vi "test - start with default path.vi"(8 "error in (no error)":errorcluster, 11 "TestCase in":refnum<class "testcase-csm-file-logger.lvclass">) -> (0 "error out":errorcluster, 3 "TestCase out":refnum<class "testcase-csm-file-logger.lvclass">)   [LabVIEW 2017, in "testcase-csm-file-logger.lvclass"]
uses:
  testcase-csm-file-logger.lvclass
  <vilib>/addons/_JKI Toolkits/VI Tester/TestCase.llb/TestCase.lvclass
  user.lib/_NEVSTOP/Communicable State Machine(CSM)/addons/Logger/CSM File Logger.lvlib
  C:/Program Files (x86)/National Instruments/LabVIEW 2017/vi.lib/addons/_JKI Toolkits/VI Tester/TestCase.llb/TestCase.lvclass
panel:
  out "LogFile":path
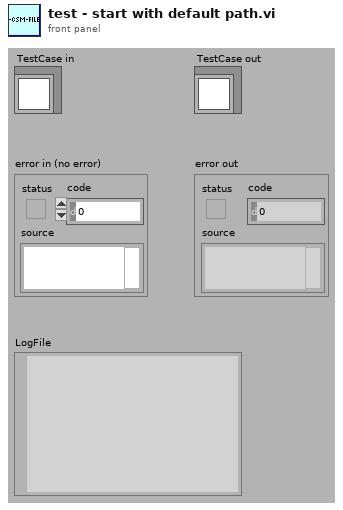
[diagram p1: front panel]
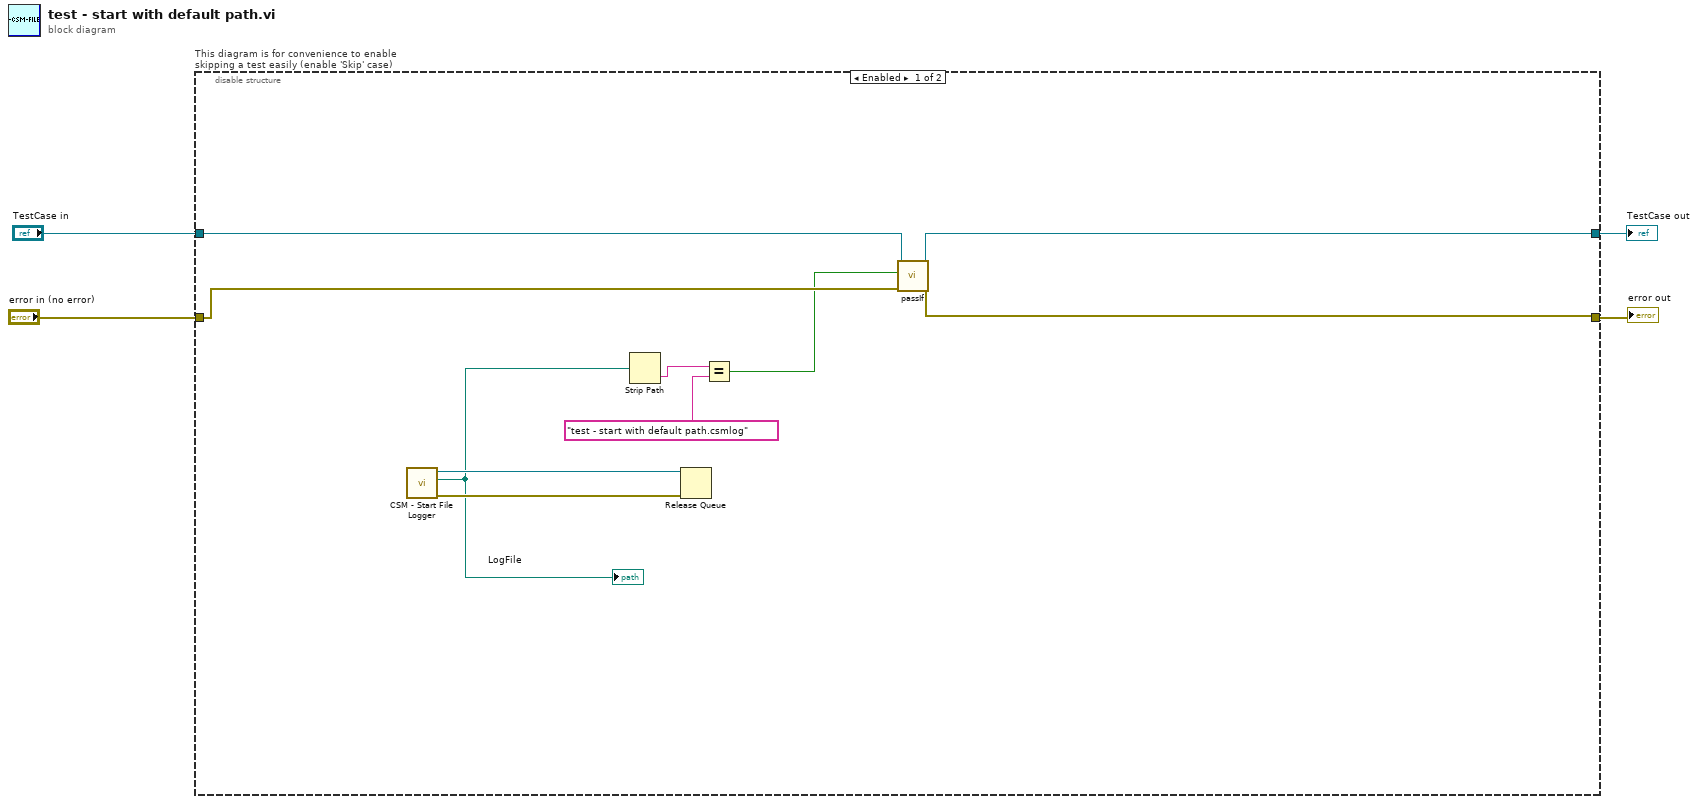
[diagram p0: block diagram]
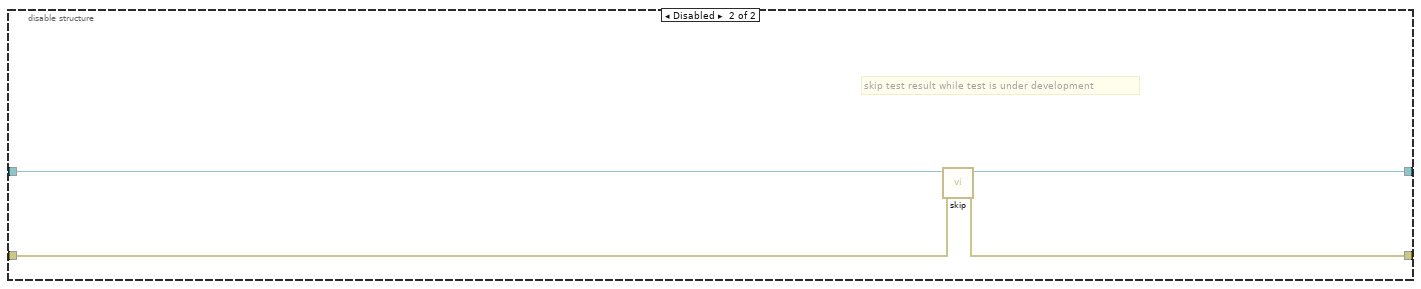
[diagram p2: hidden frame]
diagram:
  n1 = disable-structure "This diagram is for convenience to enable skipping a test easily (enable 'Skip' case)" shown="Enabled" {
    disable-tunnel: "TestCase in" -> [w14 w18]
    disable-tunnel: [w13 w16] -> w1
    disable-tunnel: [w12 w17] -> w3
    disable-tunnel: "error in (no error)" -> [w11 w15]
    frame Enabled {
      n2 = call "CSM - Start File Logger.vi"() -> ("Error out"=w9:errorcluster, "LogFile"=w8:path, "WatchDogQueue"=w10:refnum<queue>)  [unwired: 9 in]
      "LogFile" <- w8
      n3 = Strip Path(path=w8) -> (name=w7:string)  [unwired: 1 out]
      n4 = Release Queue(queue=w10, error in (no error)=w9) -> ()  [unwired: 1 in, 3 out]
      n5 = Equal?(x=w7, y="test - start with default path.csmlog") -> (x = y?=w5:bool)
      n6 = call-dynamic "passIf.vi"("error in (no error)"=w11, "pass"=w5, "TestCase in"=w14) -> ("error out"=w12:errorcluster, "TestCase out"=w13:refnum<class "testcase-csm-file-logger.lvclass">)  [unwired: 7 in]
    }
    frame Disabled {
      # "skip test result while test is under development"
      n7 = call <vilib>:"skip.vi"("error in (no error)"=w15, "TestCase in"=w18) -> ("error out"=w17:errorcluster, "TestCase out"=w16:refnum<class "testcase-csm-file-logger.lvclass">)  [unwired: 8 in]
    }
  }
  "error out" <- w3
  "TestCase out" <- w1
